vi "Labview part a.vi"() -> ()   [LabVIEW 2011]
uses:
  <vilib>/express/express analysis/Spectral/Block/exnSpectralBlock spectral measurements RMS poly.vi
  <vilib>/express/express analysis/Spectral/Block/exnSpectralBlock spectral measurements RMS DDT.vi
  <vilib>/express/express analysis/Spectral/XNode/ExpressSpectralMeasurementsBlockNode.xnode
panel:
  in  "stop":bool
  out "Fast Fourier Transform":dynamicdata(graph)
  out "Waveform Graph":dynamicdata(graph)
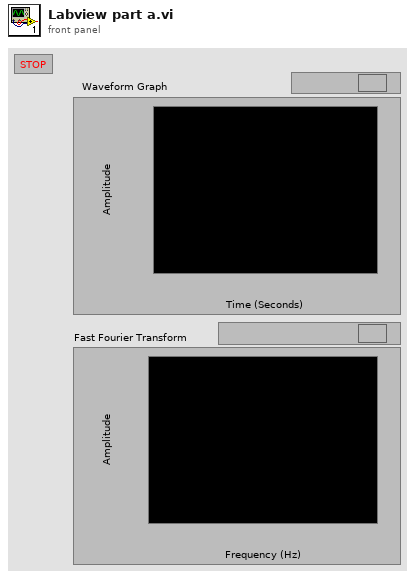
[diagram p1: front panel]
types:
  T1 = cluster{"averaging mode":u16, "weighting mode":u16, "number of averages":u32}
  T2 = cluster{"dB On (F)":bool, "unwrap phase (F)":bool, "convert to degree (F)":bool}
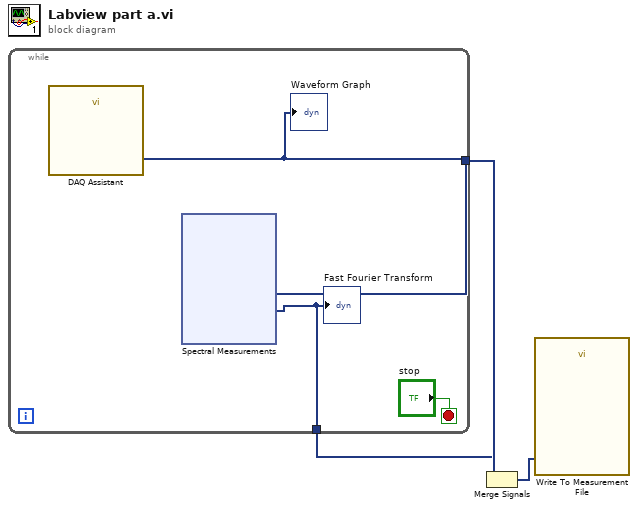
[diagram p0: block diagram]
diagram:
  n1 = while {
    tunnel: [w5] -> w3
    tunnel: [w4] -> w1
    stop <- "stop" stop-if-true
    n2 = call "DAQ Assistant"() -> ("data"=w5:dynamicdata)  [unwired: 17 in, 2 out]
    "Waveform Graph" <- w5
    n3 = xnode "Spectral Measurements"("Signals"=w5) -> ("FFT - (RMS)"=w4:dynamicdata)  [unwired: 1 in, 2 out]
    "Fast Fourier Transform" <- w4
  }
  n4 = Merge Signals(w3, w1) -> (w2:dynamicdata)
  n5 = call "Write To Measurement File"("Signals"=w2) -> ()  [unwired: 16 in, 3 out]
